vi "jettl Msg Template.vi"   [LabVIEW 2021, in "_Template.lvlib" / "Templates.lvlib" / "jettl Msg Template.lvlib"]
uses:
  jettl Msg Template.lvlib
  Template Msg Strategy/Template Msg Strategy.lvclass
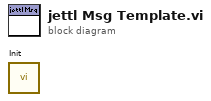
[diagram p0: block diagram]
diagram:
  n1 = call "Init.vi"() -> ()  [unwired: 11 in, 1 out]
